vi "Element Init.vi"(7 "VolatusAPI":refnum<class "VolatusAPI.lvclass">, 8 "error in (no error)":errorcluster, 10 "JSON":string, 11 "LocalGraphBuffer in":refnum<class "LocalGraphBuffer.lvclass">) -> (0 "error out":errorcluster, 3 "LocalGraphBuffer out":refnum<class "LocalGraphBuffer.lvclass">)   [LabVIEW 2020, in "VolatusGUIElements.lvlib" / "LocalGraphBuffer.lvclass"]
uses:
  LocalGraphBuffer.lvclass
  C:/dev/lv20CE/relink/lv-volatus/VolatusGUI/GUI Element/GUI Element.lvclass
  Volatus/VolatusAPI/VolatusAPI.lvclass
  JSON.ctl
  VolatusGUI/GUI Element/GUI Element.lvclass/GUI Element.ctl
  LocalGraphBuffer.lvclass/LocalGraphBuffer.ctl
  86935f47-605f-4470-b8a5-4f5d0cdfefb4.vi
  <vilib>/JDP Science/JSONtext/JSON text to Variant.vi
  <vilib>/JDP Science/JSONtext/LVClass Serializer/JSONtext LVClass Serializer.lvclass
  VolatusGUI/GUI Element/GUI Element.lvclass
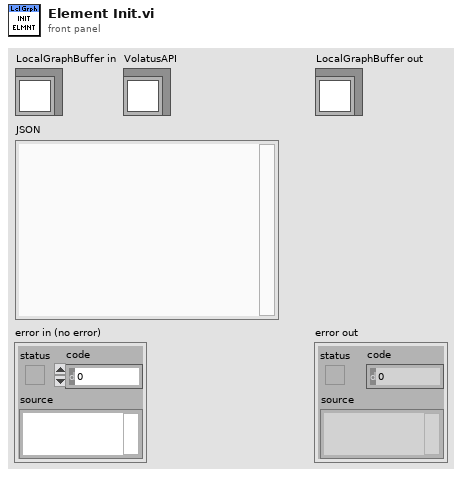
[diagram p1: front panel]
types:
  T1 = typedef "VolatusGUIElements.lvlib/LocalGraphBuffer.lvclass/JSON.ctl" = cluster{"Channels":string[], "Buffer_Length":i32, "Redraw_Period_s":dbl, "Duration_s":dbl}
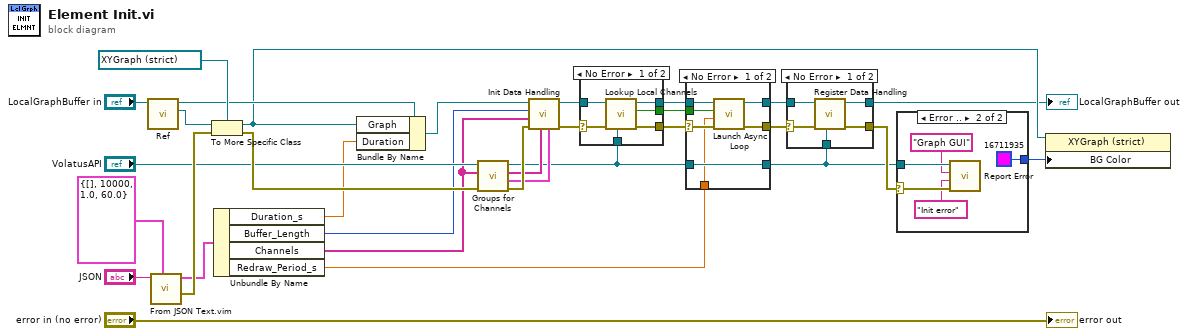
[diagram p0: block diagram]
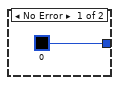
[diagram p5: hidden frame]
diagram:
  n1 = call "Ref.vi"("GUI Element in"="LocalGraphBuffer in") -> ("Ref"=w18:refnum<vi>, "GUI Element out"=w15:refnum<class "LocalGraphBuffer.lvclass">)  [unwired: 9 in]
  n2 = call "From JSON Text.vim"("Data Type and Default Value"=T1 {"Channels"=[], "Buffer_Length"=10000, "Redraw_Period_s"=1.0, "Duration_s"=60.0} ("JSON"), "JSON"="JSON") -> ("error out"=w30:errorcluster, "Data out"=w20:T1)  [unwired: 8 in]
  n3 = To More Specific Class(target class=refnum<vi> refnum ("XY Graph"), reference=w18, error in=w30) -> (specific class reference=w13:refnum<vi>, error out=w31:errorcluster)
  n4 = Unbundle By Name(w20) -> ("Duration_s"=w9:dbl, "Buffer_Length"=w21:i32, "Channels"=w22:string[], "Redraw_Period_s"=w19:dbl)
  n5 = Bundle By Name(cluster=w15, "Graph"=w13, "Duration"=w9) -> (w12:refnum<class "LocalGraphBuffer.lvclass">)
  n6 = call "Groups for Channels.vi"("error in (no error)"=w31, "Channels"=w22, "VolatusAPI in"="VolatusAPI") -> ("error out"=w29:errorcluster, "Channels per Group"=w23:cluster{cluster{"Index":i32, "Name":string}[]}[], "Groups"=w24:string[], "VolatusAPI out"=w6:refnum<class "VolatusAPI.lvclass">)  [unwired: 5 in]
  n7 = call "Init Data Handling.vi"("Channels per Group"=w23, "Groups"=w24, "error in (no error)"=w29, "Channels"=w22, "Buffer Size"=w21, "LocalGraphBuffer in"=w12) -> ("error out"=w8:errorcluster, "LocalGraphBuffer out"=w7:refnum<class "LocalGraphBuffer.lvclass">)  [unwired: 4 in]
  n8 = case shown="No Error" w8 {
    selector: w8 -> [w36 w39]
    tunnel: w7 -> [w38 w40]
    tunnel: [w37 w40] -> w4
    tunnel: [w35 w39] -> w5
    tunnel: w6 -> [w34 _]
    tunnel: [w33 _] -> w1
    frame No Error {
      n9 = call "Lookup Local Channels.vi"("VolatusAPI"=w34, "error in (no error)"=w36, "LocalGraphBuffer in"=w38) -> ("error out"=w35:errorcluster, "Has Local"=w33:bool, "LocalGraphBuffer out"=w37:refnum<class "LocalGraphBuffer.lvclass">)  [unwired: 6 in]
    }
    frame Error {
    }
  }
  n10 = case shown="No Error" w5 {
    selector: w5 -> [w43 w50]
    tunnel: w4 -> [w47 w49]
    tunnel: w6 -> [w44 w48]
    tunnel: [w46 w49] -> w10
    tunnel: w19 -> [w42 _]
    tunnel: [w45 w50] -> w11
    tunnel: [w44 w48] -> w3
    tunnel: w1 -> [w41 _]
    frame No Error {
      n11 = call "Launch Async Loop.vi"("error in (no error)"=w43, "Redraw Period"=w42, "Has Local"=w41, "LocalGraphBuffer in"=w47) -> ("error out"=w45:errorcluster, "LocalGraphBuffer out"=w46:refnum<class "LocalGraphBuffer.lvclass">)  [unwired: 6 in]
    }
    frame Error {
    }
  }
  n12 = case shown="No Error" w11 {
    selector: w11 -> [w54 w56]
    tunnel: w10 -> [w55 w57]
    tunnel: [w53 w57] -> w2
    tunnel: [w52 w56] -> w32
    tunnel: w3 -> [w51 _]
    frame No Error {
      n13 = call "Register Data Handling.vi"("VolatusAPI in"=w51, "error in (no error)"=w54, "LocalGraphBuffer in"=w55) -> ("error out"=w52:errorcluster, "LocalGraphBuffer out"=w53:refnum<class "LocalGraphBuffer.lvclass">)  [unwired: 7 in]
    }
    frame Error {
    }
  }
  "LocalGraphBuffer out" <- w2
  n14 = case shown="Error .." w32 {
    selector: w32 -> [_ w62]
    tunnel: w3 -> [_ w63]
    tunnel: [u32 0 ("Plot Area:Colors:BG Color") u32 16711935 ("Plot Area:Colors:BG Color")] -> w14
    frame No Error {
    }
    frame Error {
      n15 = call "Report Error.vi"("error in (no error)"=w62, "Message"="Init error" ("Context"), "Context"="Graph GUI", "VolatusAPI in"=w63) -> ()  [unwired: 6 in, 2 out]
    }
  }
  n16 = property class="XYGraph (strict)"(reference=w13, "BG Color"=w14) -> ()  [unwired: 1 in, 2 out]
  "error out" <- "error in (no error)"
